vi "LeerCorriente_Ini.vi"() -> (0 "error out":errorcluster, 1 "output cluster":T1)   [LabVIEW 2017]
uses:
  <vilib>/DAQmx/create/channels.llb/DAQmx Create Channel (AI-Voltage-Basic).vi
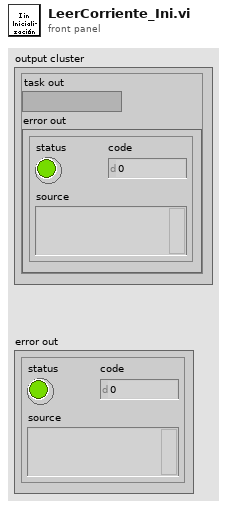
[diagram p1: front panel]
types:
  T1 = cluster{"task out":refnum<k21>, "error out":errorcluster}
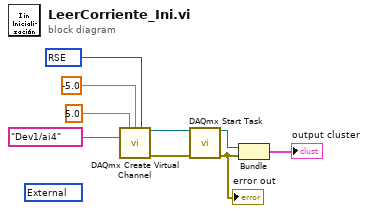
[diagram p0: block diagram]
diagram:
  (unwired) 10167 items=["default"=-1, "Internal"=10200, "External"=10167] ("shunt resistor location")
  w2 = 10083 items=["Default"=-1, "RSE"=10083, "Differential"=10106, "Pseudodifferential"=12529] ("output terminal configuration")
  n1 = call-poly <vilib>:"DAQmx Create Virtual Channel.vi"("maximum value"=5.0, "minimum value"=-5.0, "input terminal configuration"=w2, "physical channels"=tag "Dev1/ai4") -> ("task out"=w6:refnum<k21>, "error out"=w5:errorcluster)  [unwired: 10 in]
  n2 = call <vilib>:"DAQmx Start Task.vi"("task/channels in"=w6, "error in"=w5) -> ("task out"=w8:refnum<k21>, "error out"=w9:errorcluster)  [unwired: 12 in]
  "error out" <- w9
  n3 = Bundle("task out"=w8, "error out"=w9) -> (→"output cluster":T1)  [unwired: 1 in]
